vi "ErrorLog.vi"(9 "error in (no error)":errorcluster, 10 "Step No.":string) -> (1 "error out":errorcluster)   [LabVIEW 2013]
uses:
  Control/Buffer.vi
panel:
  out "created path":path
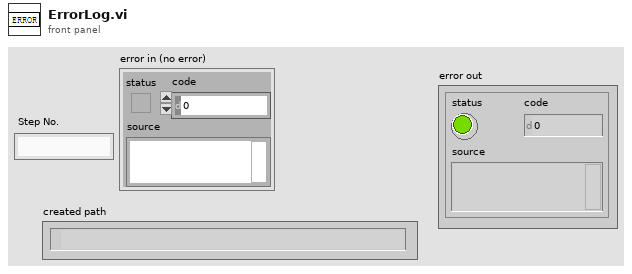
[diagram p1: front panel]
types:
  T1 = enum16{"open", "replace", "create", "open or create", "replace or create", "replace or create with confirmation"}
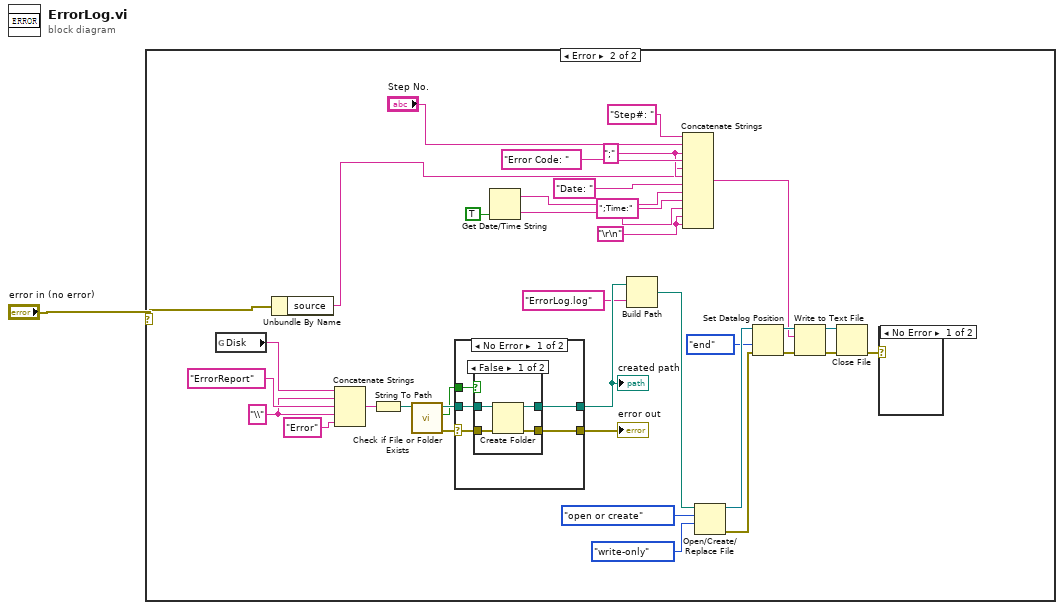
[diagram p0: block diagram]
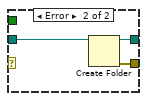
[diagram p5: hidden frame]
diagram:
  n1 = case shown="Error" "error in (no error)" {
    selector: "error in (no error)" -> [_ w3]
    frame No Error {
    }
    frame Error {
      w4 = "\r\n"
      w10 = ";" ("string")
      w30 = "\\" ("string")
      n2 = global read "Buffer.vi" "Disk"() -> (w29:string)
      n3 = Unbundle By Name(w3) -> ("source"=w2:string)
      n4 = Concatenate Strings(w29, w30, "ErrorReport" ("string"), w30, "Error" ("string")) -> (w32:string)
      n5 = String To Path(string=w32) -> (path=w36:path)
      n6 = call <vilib>:"Check if File or Folder Exists.vi"("path"=w36) -> ("error out"=w33:errorcluster, "file or folder exists?"=w34:bool, "dup path"=w35:path)  [unwired: 8 in]
      n7 = case shown="No Error" w33 {
        selector: w33 -> [w39 _]
        tunnel: w35 -> [w42 w51]
        tunnel: w34 -> [w41 _]
        tunnel: [w40 w50] -> w17
        tunnel: [w38 w49] -> w37
        frame No Error {
          n8 = case shown="False" w41 {
            tunnel: w42 -> [w46 w48]
            tunnel: [w45 w48] -> w40
            tunnel: w39 -> [w44 w47]
            tunnel: [w43 w47] -> w38
            frame False {
              n9 = Create Folder(path (use dialog)=w46, error in=w44) -> (created path=w45:path, error out=w43:errorcluster)  [unwired: 1 in, 1 out]
            }
            frame True {
            }
          }
        }
        frame Error {
          n10 = Create Folder(path (use dialog)=w51) -> (created path=w50:path, error out=w49:errorcluster)  [unwired: 2 in, 1 out]
        }
      }
      "error out" <- w37
      "created path" <- w17
      n11 = Get Date/Time String(want seconds? (F)=TRUE) -> (date string=w8:string, time string=w6:string)  [unwired: 2 in]
      n12 = Build Path(base path=w17, name or relative path="ErrorLog.log") -> (appended path=w16:path)
      n13 = Concatenate Strings("Step#: " ("string"), "Step No.", w10, "Error Code: " ("string"), w2, w10, "Date: " ("string"), w8, ";Time:" ("string"), w6, w4, w4) -> (w14:string)
      n14 = Open/Create/Replace File(file path (use dialog)=w16, operation (0:open)=T1."open or create", access (0:read/write)=enum16{"read/write", "read-only", "write-only"}."write-only") -> (refnum out=w23:refnum<file>, error out=w21:errorcluster)  [unwired: 3 in, 1 out]
      n15 = Set Datalog Position(4:w21, 5:enum16{"start", "end", "current"}."end" ("from (0:start)"), 7:w23) -> (0:w19:errorcluster, 3:w22:refnum<file>)  [unwired: 1 in]
      n16 = Write to Text File(file (use dialog)=w22, text=w14, error in=w19) -> (refnum out=w27:refnum<file>, error out=w26:errorcluster)  [unwired: 1 in, 1 out]
      n17 = Close File(refnum=w27, error in=w26) -> (error out=w18:errorcluster)  [unwired: 1 out]
      n18 = case shown="No Error" w18 {
        frame No Error {
        }
        frame Error {
        }
      }
    }
  }
